vi "SetControl_EIP.vi"(10 "Boolean array 2":bool[][](array[boolean]), 11 "variant":T1) -> (3 "Data":u8[](array[numeric]) format="%x")   [LabVIEW 2014]
uses:
  Control_EIP.ctl
panel:
  out "Boolean array":bool[][](array[boolean])
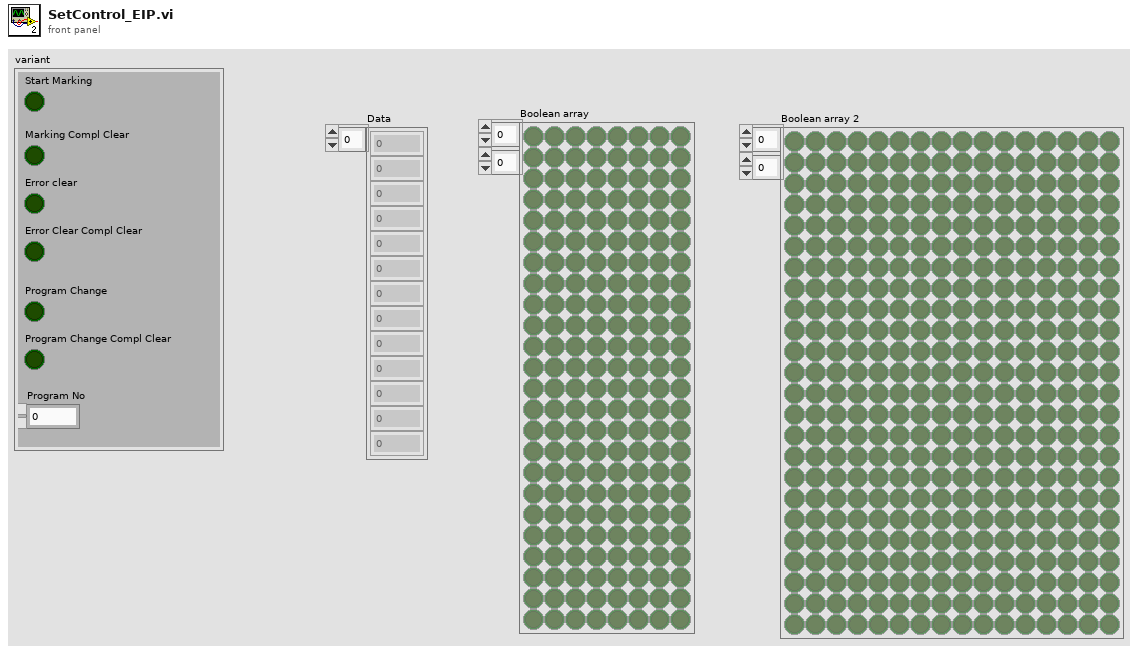
[diagram p1: front panel]
types:
  T1 = typedef "Control_EIP.ctl" = cluster{"Start Marking":bool, "Error clear":bool, "Program Change":bool, "Marking Compl Clear":bool, "Program No":u16, "Error Clear Compl Clear":bool, "Program Change Compl Clear":bool}
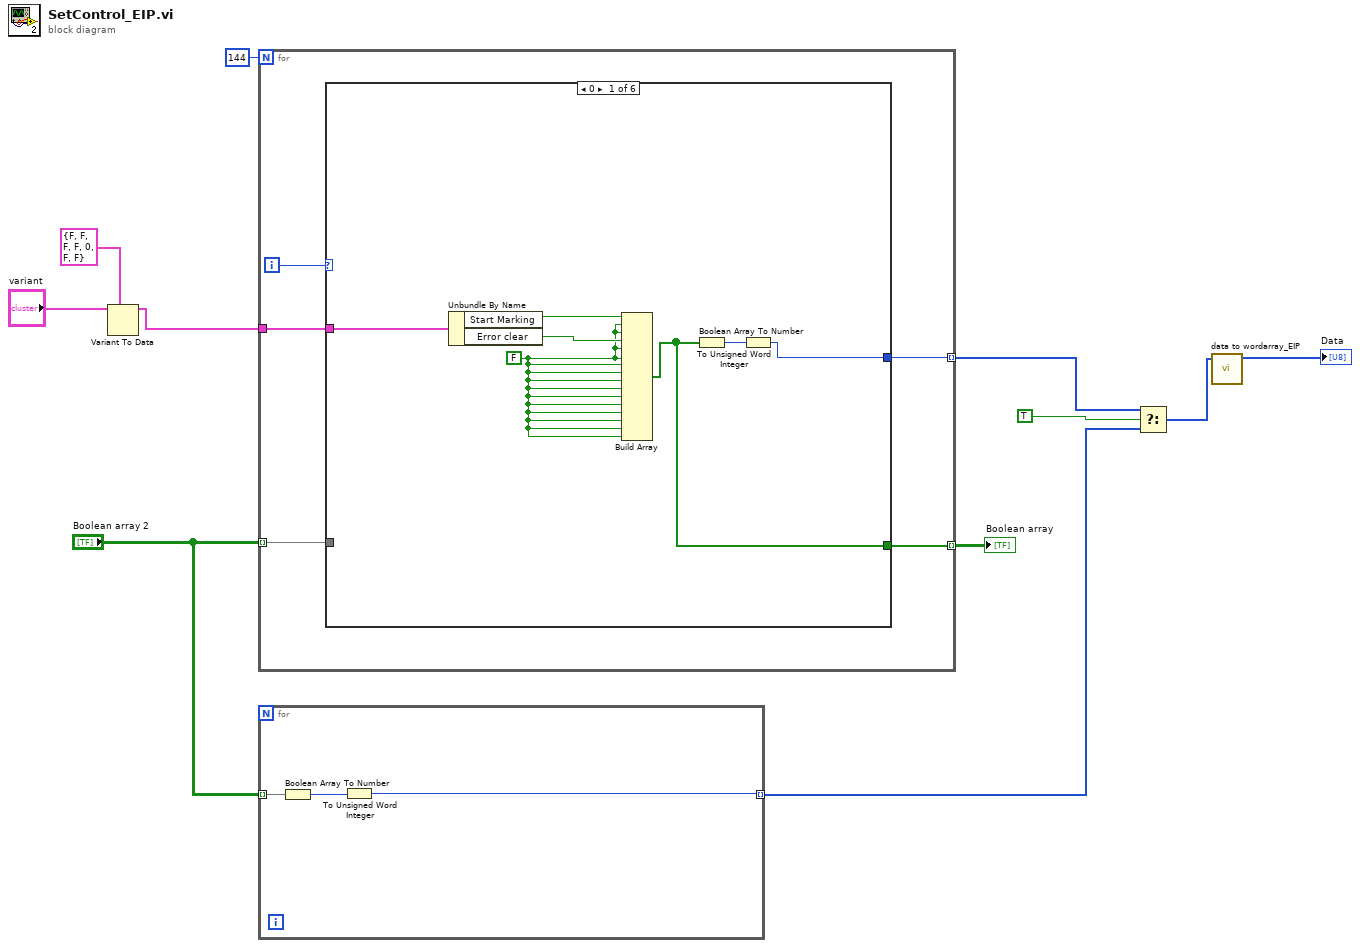
[diagram p0: block diagram]
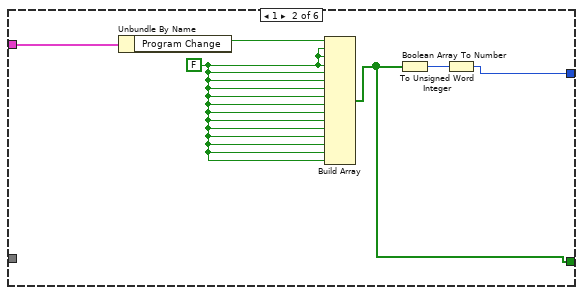
[diagram p2: hidden frame]
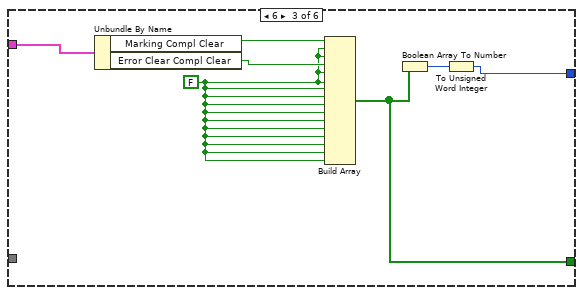
[diagram p3: hidden frame]
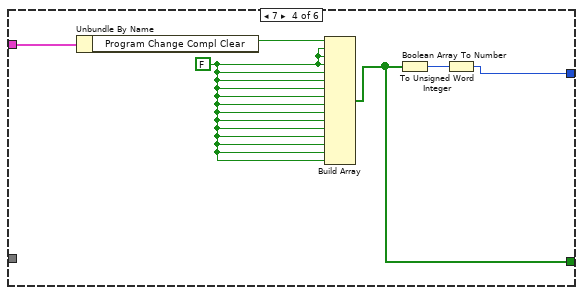
[diagram p4: hidden frame]
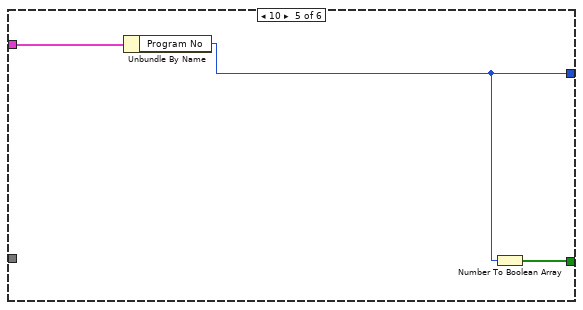
[diagram p5: hidden frame]
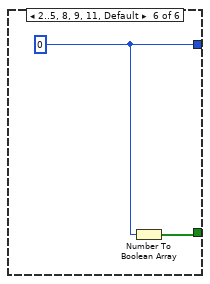
[diagram p6: hidden frame]
diagram:
  n1 = Variant To Data(type=T1 {"Start Marking"=FALSE, "Error clear"=FALSE, "Program Change"=FALSE, "Marking Compl Clear"=FALSE, "Program No"=0, "Error Clear Compl Clear"=FALSE, "Program Change Compl Clear"=FALSE}, Variant="variant") -> (data=w9:T1)  [unwired: 1 in, 1 out]
  n2 = for {
    N: 144 -> [_]
    tunnel: [w14] -> w4 mode=indexing
    tunnel: w9 -> [w15]
    tunnel: [w13] -> w6 mode=indexing
    tunnel: "Boolean array 2" -> [w12] mode=indexing
    i -> [w16]
    n3 = case shown="0" w16 {
      tunnel: [w19 w26 w33 w38 w43 w47] -> w14
      tunnel: w15 -> [w21 w27 w34 w40 w45 _]
      tunnel: [w17 w24 w30 w37 w44 w46] -> w13
      tunnel: w12 -> [_ _ _ _ _ _]
      frame 0 {
        w18 = FALSE ("element")
        n4 = Unbundle By Name(w21) -> ("Start Marking"=w23:bool, "Error clear"=w20:bool)
        n5 = Build Array(w23, w18, w18, w20, w18, w18, w18, w18, w18, w18, w18, w18, w18, w18, w18, w18) -> (w17:bool[])
        n6 = Boolean Array To Number(Boolean array=w17) -> (number=w22:u32)
        n7 = To Unsigned Word Integer(number=w22) -> (unsigned 16bit integer=w19:u16)
      }
      frame 1 {
        w25 = FALSE ("element")
        n8 = Unbundle By Name(w27) -> ("Program Change"=w28:bool)
        n9 = Build Array(w28, w25, w25, w25, w25, w25, w25, w25, w25, w25, w25, w25, w25, w25, w25, w25) -> (w24:bool[])
        n10 = Boolean Array To Number(Boolean array=w24) -> (number=w29:u32)
        n11 = To Unsigned Word Integer(number=w29) -> (unsigned 16bit integer=w26:u16)
      }
      frame 6 {
        w31 = FALSE ("element")
        n12 = Unbundle By Name(w34) -> ("Marking Compl Clear"=w35:bool, "Error Clear Compl Clear"=w32:bool)
        n13 = Build Array(w35, w31, w31, w32, w31, w31, w31, w31, w31, w31, w31, w31, w31, w31, w31, w31) -> (w30:bool[])
        n14 = Boolean Array To Number(Boolean array=w30) -> (number=w36:u32)
        n15 = To Unsigned Word Integer(number=w36) -> (unsigned 16bit integer=w33:u16)
      }
      frame 7 {
        w39 = FALSE ("element")
        n16 = Unbundle By Name(w40) -> ("Program Change Compl Clear"=w41:bool)
        n17 = Build Array(w41, w39, w39, w39, w39, w39, w39, w39, w39, w39, w39, w39, w39, w39, w39, w39) -> (w37:bool[])
        n18 = Boolean Array To Number(Boolean array=w37) -> (number=w42:u32)
        n19 = To Unsigned Word Integer(number=w42) -> (unsigned 16bit integer=w38:u16)
      }
      frame 10 {
        n20 = Unbundle By Name(w45) -> ("Program No"=w43:u16)
        n21 = Number To Boolean Array(number=w43) -> (Boolean array=w44:bool[])
      }
      frame 2..5, 8, 9, 11, Default {
        w47 = u16 0
        n22 = Number To Boolean Array(number=w47) -> (Boolean array=w46:bool[])
      }
    }
  }
  "Boolean array" <- w6
  n23 = for {
    tunnel: "Boolean array 2" -> [w50] mode=indexing
    tunnel: [w48] -> w3 mode=indexing
    n24 = Boolean Array To Number(Boolean array=w50) -> (number=w49:u32)
    n25 = To Unsigned Word Integer(number=w49) -> (unsigned 16bit integer=w48:u16)
  }
  n26 = Select(t=w4, s=TRUE, f=w3) -> (s? t:f=w2:u16[])
  n27 = call "data to wordarray_EIP.vi"("Data"=w2) -> ("Word array"=→"Data":u16[])  [unwired: 10 in]
